vi "Power Meter Control Panel.vi"(8 "error in (no error)":errorcluster) -> (0 "error out":errorcluster)   [LabVIEW 2013]
doc: "(Dynamic) A user-level application that simulates the physical front panel of the Instrument. Provide the user with buttons to manually control features of the instrument, and provide indicators of its current state."
uses:
  Public/Filters.ctl
  <vilib>/Instr/_visa.llb/VISA Configure Serial Port (Instr).vi
  Newport 1830-C.lvlib
panel:
  in  "Baud rate (9600)":u32=115200
  out "Waveform Chart":dbl[unit](graph)=4.09e-07
  out "Sampling Rate":dbl
  in  "Which Filter":T1=1 items=["Orange"=1, "Green"=2, "Yellow"=3]
  out "Actual Power":dbl
  in  "Measured Power":dbl
  in  "Convert Power":bool
  in  "VISA Resource Name":refnum<visa-resource-name>="COM10"
  out "Initialized?":bool
  in  "Filter":T1=1 items=["Orange"=1, "Green"=2, "Yellow"=3]
  out "Power":string
  in  "Time between Reads (ms)":u32 max=1000 step=1
  in  "Read Continuous":bool
  in  "Averaging":u32=40 min=1 max=1024 step=1
  in  "Averaging":bool
  out "Units":u16(ring)=1 items=["W"=1, "dB"=2, "dBm"=3, "REL"=4]
  out "AVG":u16(ring)=2 items=["Slow"=1, "Medium"=2, "Fast"=3]
  out "Run/Stop":u16(ring) items=["Stop", "Run"]
  out "ATTN":u16(ring) items=["Off", "On"]
  out "Local Lockout":u16(ring) items=["Off", "On"]
  out "Zero":u16(ring) items=["Off", "On"]
  out "Beeper":u16(ring) items=["Off", "On"]
  out "Backlight":u16(ring) items=["Off", "Low", "High"]
  out "Range":u16(ring) items=["Auto", "Highest Sensitivity", "30uW", "300uW", "3mW", "30mW", "300mW", "3W", "Lowest Sensitivity"]
  in  "Run/Stop set":u32(ring)=1 items=["Stop", "Run"]
  in  "ATTN set":u32(ring) items=["Off", "On"]
  in  "BKLT set":u32(ring)=1 items=["Off", "Low", "High"]
  in  "Range set":u32(ring) items=["Auto", "Highest Sensitivity", "30uW", "300uW", "3mW", "30mW", "300mW", "3W", "Lowest Sensitivity"]
  in  "Beeper set":u32(ring) items=["Off", "On"]
  in  "AVG set":u32(ring)=2 items=["Slow"=1, "Medium"=2, "Fast"=3]
  in  "Units set":u32(ring)=1 items=["W"=1, "dB"=2, "mdB"=3, "REL"=4]
  in  "Zero set":u32(ring) items=["Off", "On"]
  in  "Local set":u32(ring) items=["Off", "On"]
  in  "Read Current Power":bool
  in  "Apply \nNew Settings":bool
  in  "Copy \nCurrent Settings\nto New Settings":bool
  in  "Read Settings":bool
  in  "Wavelength Set":dbl[unit]
  out "Wavelength":dbl[unit]
  in  "Copy actual to set":bool
  in  "Populate fields with member data":bool
  in  "stop":bool
  # "Newport 1830 Power Meter"
  # "New Settings"
  # "Current Settings"
  # "Convert Measured Power"
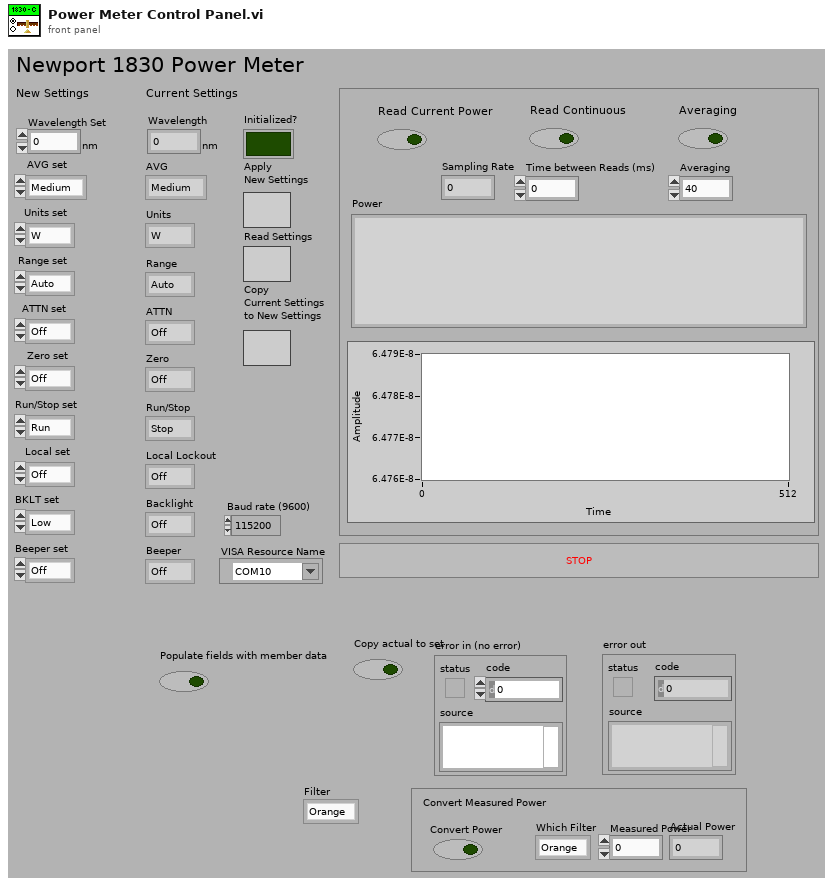
[diagram p1: front panel]
types:
  T1 = typedef "Newport 1830-C.lvlib/Filters.ctl" = u16
  T2 = cluster{"Wavelength":dbl[unit], "AVG":u16, "Range":u16, "Backlight":u16, "Beeper":u16, "Zero":u16, "Local Lockout":u16, "ATTN":u16, "Run/Stop":u16, "Units":u16, "Averaging Time":dbl, "Averaging":bool, "Most Recent Power":dbl, "Filter":T1}
  T3 = cluster{"Wavelength":dbl[unit], "AVG":u16, "Range":u16, "Backlight":u16, "Beeper":u16, "Zero":u16, "Local Lockout":u16, "ATTN":u16, "Run/Stop":u16, "Units":u16, "Averaging Points":u32, "Averaging":bool, "Most Recent Power":dbl, "Filter":T1}
  T4 = cluster{"Wavelength":dbl[unit], "AVG":i32, "Range":i32, "Backlight":i32, "Beeper":i32, "Zero":i32, "Local Lockout":i32, "ATTN":i32, "Run/Stop":i32, "Units":i32, "Averaging Points":u32, "Averaging":bool, "Most Recent Power":dbl, "Filter":i32}
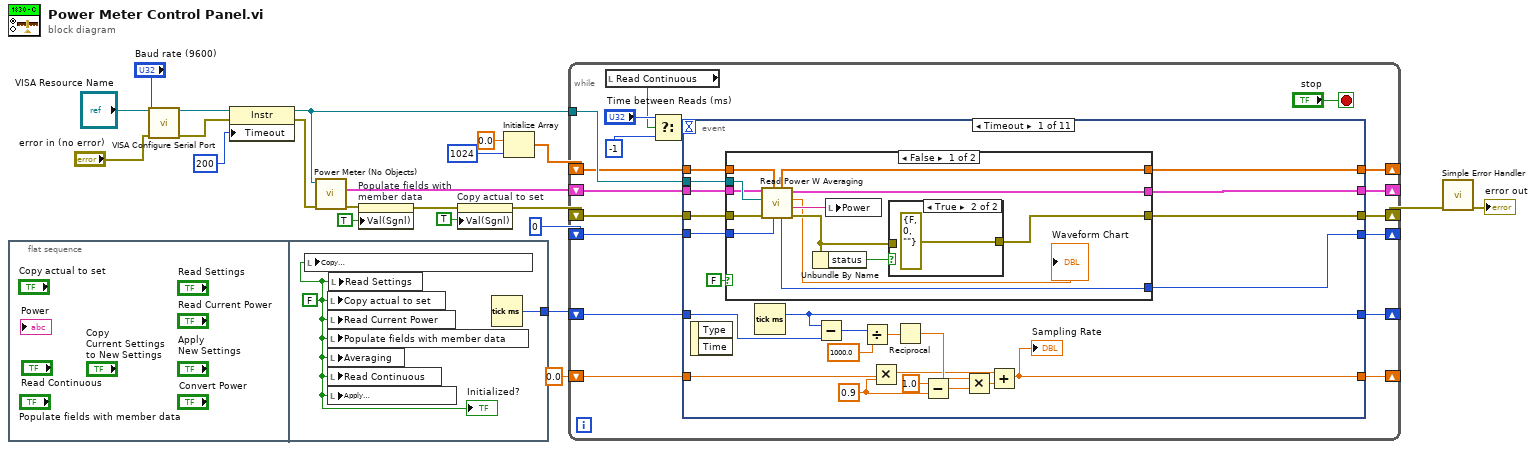
[diagram p0: block diagram]
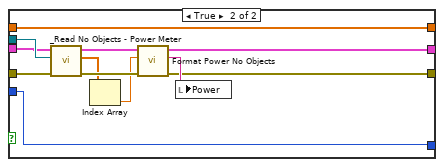
[diagram p3: hidden frame]
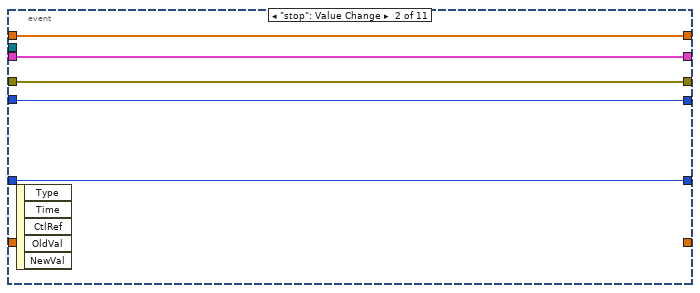
[diagram p4: hidden frame]
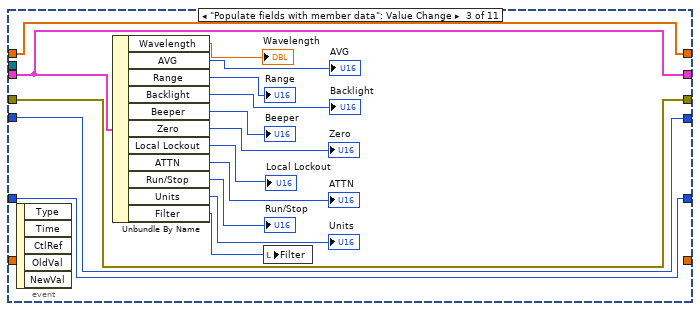
[diagram p5: hidden frame]
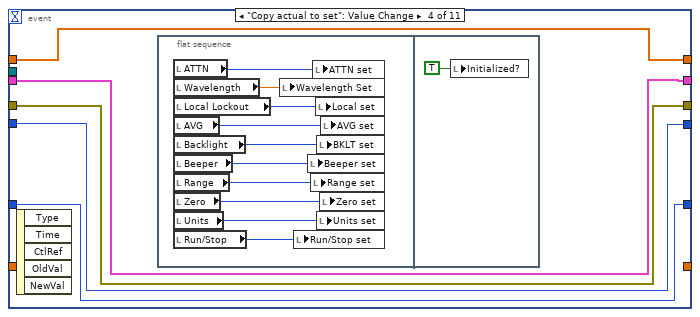
[diagram p6: hidden frame]
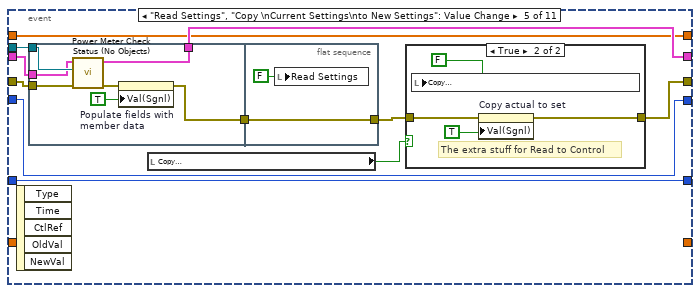
[diagram p7: hidden frame]
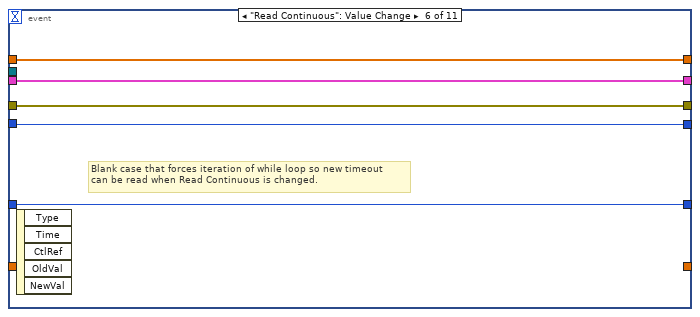
[diagram p9: hidden frame]
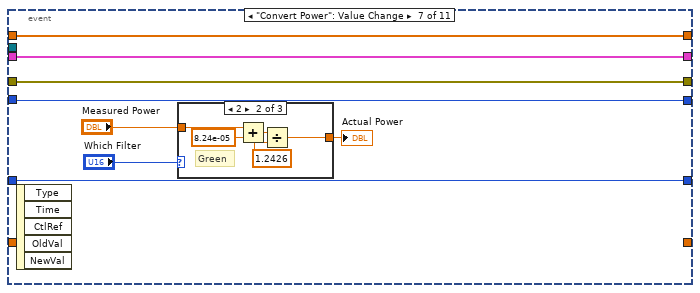
[diagram p10: hidden frame]
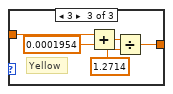
[diagram p12: hidden frame]
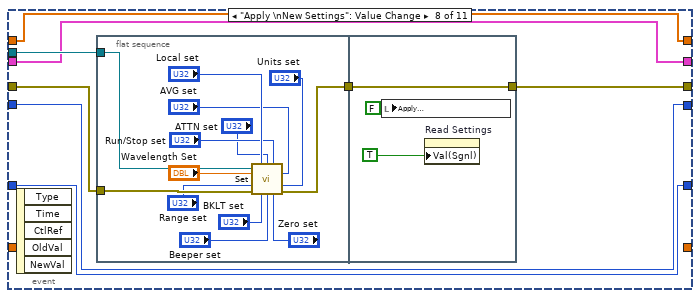
[diagram p13: hidden frame]
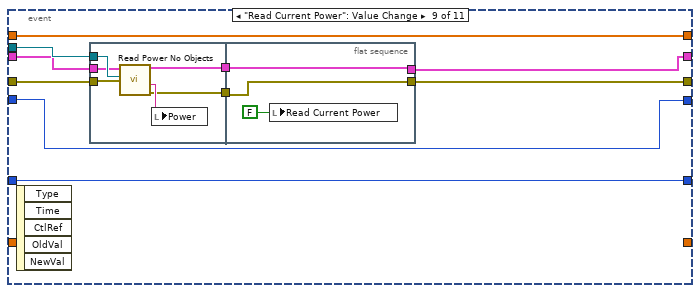
[diagram p14: hidden frame]
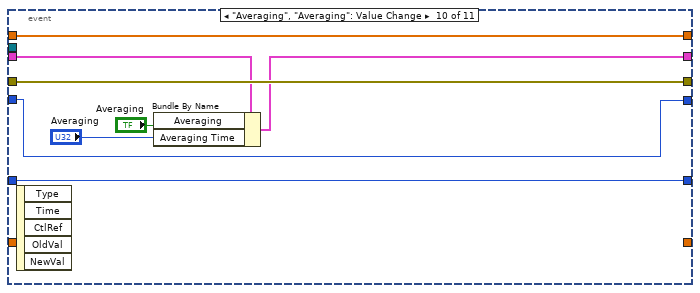
[diagram p15: hidden frame]
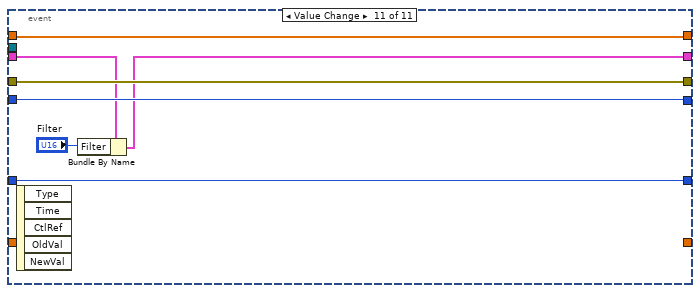
[diagram p16: hidden frame]
diagram:
  n1 = flat-sequence {
    tunnel: [w23] -> w3
    frame #0 {
    }
    frame #1 {
      w24 = FALSE ("Read")
      n2 = local write "Copy \nCurrent Settings\nto New Settings"(w24) -> ()
      n3 = local write "Copy actual to set"(w24) -> ()
      n4 = local write "Read Current Power"(w24) -> ()
      n5 = local write "Populate fields with member data"(w24) -> ()
      n6 = local write "Averaging"(w24) -> ()
      n7 = local write "Read Continuous"(w24) -> ()
      n8 = local write "Apply \nNew Settings"(w24) -> ()
      n9 = local write "Read Settings"(w24) -> ()
      n10 = Tick Count (ms)() -> (millisecond timer value=w23:u32)
      "Initialized?" <- w24
    }
  }
  n11 = call-poly "VISA Configure Serial Port"("VISA resource name"="VISA Resource Name", "baud rate (9600)"="Baud rate (9600)", "error in (no error)"="error in (no error)") -> ("VISA resource name out"=w8:refnum<visa-resource-name>, "error out"=w4:errorcluster)  [unwired: 7 in, 4 out]
  n12 = property class="Instr"(reference=w8, error in=w4, "Timeout"=u32 200 ("General Settings:Timeout Value")) -> (reference out=w9:refnum<visa-resource-name>, error out=w5:errorcluster)
  n13 = call "Power Meter (No Objects).vi"("error in (no error)"=w5, "VISA resource name"=w9) -> ("error out"=w16:errorcluster, "Power Meter Out"=w11:T2)  [unwired: 8 in]
  n14 = property on="Populate fields with member data" class="Bool (strict)"(error in=w16, "Val(Sgnl)"=TRUE ("Value (Signaling)")) -> (error out=w20:errorcluster)  [unwired: 1 in, 1 out]
  n15 = property on="Copy actual to set" class="Bool (strict)"(error in=w20, "Val(Sgnl)"=TRUE ("Value (Signaling)")) -> (error out=w19:errorcluster)  [unwired: 1 in, 1 out]
  n16 = Initialize Array(0.0 ("element"), 1024 ("dimension size")) -> (w13:dbl[])
  n17 = while {
    shift-right: [w41] -> _
    shift-left: w11 -> [w27]
    shift-right: [w40] -> w18
    shift-left: w19 -> [w42]
    tunnel: w9 -> [w37]
    shift-right: [w32] -> _
    shift-left: w13 -> [w33]
    shift-right: [w30] -> _
    shift-left: 0 -> [w31]
    shift-right: [w29] -> _
    shift-left: w3 -> [w28]
    shift-right: [w26] -> _
    shift-left: 0.0 -> [w25]
    stop <- "stop" stop-if-true
    n18 = local read "Read Continuous"() -> (w35:bool)
    n19 = Select(t="Time between Reads (ms)", s=w35, f=-1) -> (s? t:f=w38:u32)
    n20 = event shown="[0] Timeout" {
      selector: _ -> [_ _ _ _ _ _ _ _ _ _ _]
      dyn-events: _ -> [_ _ _ _ _ _ _ _ _ _ _]
      timeout: w38 -> [_ _ _ _ _ _ _ _ _ _ _]
      tunnel: [w61 w94 w98 w114 w135 w157 w160 w179 w207 w224 w230] -> w41
      tunnel: [w64 w97 w112 w118 w136 w159 w167 w185 w209 w229 w235] -> w40
      tunnel: w42 -> [w65 w97 w112 w118 w140 w159 w167 w186 w211 w229 w235]
      tunnel: w37 -> [w63 _ _ _ w134 _ _ w184 w208 _ _]
      tunnel: w33 -> [w60 w96 w101 w117 w133 w158 w163 w182 w206 w226 w234]
      tunnel: [w59 w96 w101 w117 w133 w158 w163 w182 w206 w226 w234] -> w32
      tunnel: w31 -> [w58 w93 w99 w116 w131 w155 w161 w180 w204 w222 w232]
      tunnel: [w57 w93 w99 w116 w131 w155 w161 w180 w204 w222 w232] -> w30
      tunnel: [w55 w95 w100 w115 w130 w156 w162 w181 w203 w223 w233] -> w29
      tunnel: w28 -> [w56 w95 w100 w115 w130 w156 w162 w181 w203 w223 w233]
      tunnel: w27 -> [w52 w94 w98 w114 w132 w157 w160 w179 w205 w225 w231]
      tunnel: [w43 _ _ _ _ _ _ _ _ _ _] -> w26
      tunnel: w25 -> [w51 _ _ _ _ _ _ _ _ _ _]
      event Timeout {
        w48 = 0.9 ("y")
        n21 = event-data() -> ()  [unwired: 1 in, 2 out]
        n22 = case shown="False" FALSE {
          tunnel: w65 -> [w77 w92]
          tunnel: [w72 w87] -> w64
          tunnel: [w76 w86] -> w61
          tunnel: w63 -> [w78 w85]
          tunnel: w60 -> [w71 w83]
          tunnel: [w70 w83] -> w59
          tunnel: w58 -> [w69 w82]
          tunnel: [w68 w82] -> w57
          tunnel: w52 -> [w66 w81]
          frame False {
            n23 = call "Read Power W Averaging.vi"("Index In"=w69, "Buffer In"=w71, "error in (no error)"=w77, "VISA Resource Name"=w78, "Cluster In"=w66) -> ("error out"=w74:errorcluster, "Current Power w/ Units"=w75:string, "Current Power"=→"Waveform Chart":dbl[unit], "Cluster Out"=w76:T3, "Index Out"=w68:u32, "Buffer Out"=w70:dbl[])  [unwired: 1 in]
            n24 = Unbundle By Name(w74) -> ("status"=w73:bool)
            n25 = local write "Power"(w75) -> ()
            n26 = case shown="True" w73 {
              tunnel: w74 -> [w79 _]
              tunnel: [w79 errorcluster {"status"=FALSE, "code"=0, "source"=""} ("error out")] -> w72
              frame False {
              }
              frame True {
              }
            }
          }
          frame True {
            n27 = call "_Read No Objects - Power Meter.vi"("error in (no error)"=w92, "VISA Resource Name In"=w85, "Power Meter in"=w81) -> ("error out"=w91:errorcluster, "X array"=w90:dbl[], "Power Meter Out"=w84:T4)  [unwired: 5 in, 1 out]
            n28 = Index Array(array=w90) -> (element=w89:dbl)  [unwired: 1 in]
            n29 = call "Format Power No Objects.vi"("error in"=w91, "Power"=w89, "Cluster In"=w84) -> ("error out"=w87:errorcluster, "Formatted Power"=w88:string, "Cluster Out"=w86:T3)  [unwired: 6 in]
            n30 = local write "Power"(w88) -> ()
          }
        }
        n31 = Tick Count (ms)() -> (millisecond timer value=w55:u32)
        n32 = Subtract(x=w55, y=w56) -> (x-y=w54:u32)
        n33 = Divide(x=w54, y=1000.0) -> (x/y=w53:dbl)
        n34 = Multiply(x=w51, y=w48) -> (x*y=w44:dbl)
        n35 = Reciprocal(x=w53) -> (1/x=w50:dbl)
        n36 = Subtract(x=1.0, y=w48) -> (x-y=w46:dbl)
        n37 = Multiply(x=w50, y=w46) -> (x*y=w45:dbl)
        n38 = Add(x=w44, y=w45) -> (x+y=w43:dbl)
        "Sampling Rate" <- w43
      }
      event "stop": Value Change {
        n39 = event-data() -> ()  [unwired: 1 in, 5 out]
      }
      event "Populate fields with member data": Value Change {
        n40 = event-data() -> ()  [unwired: 1 in, 5 out]
        n41 = Unbundle By Name(w98) -> ("Wavelength"=→"Wavelength":dbl[unit], "AVG"=→"AVG":u16, "Range"=→"Range":u16, "Backlight"=→"Backlight":u16, "Beeper"=→"Beeper":u16, "Zero"=→"Zero":u16, "Local Lockout"=→"Local Lockout":u16, "ATTN"=→"ATTN":u16, "Run/Stop"=→"Run/Stop":u16, "Units"=→"Units":u16, "Filter"=w102:T1)
        n42 = local write "Filter"(w102) -> ()
      }
      event "Copy actual to set": Value Change {
        n43 = event-data() -> ()  [unwired: 1 in, 5 out]
        n44 = flat-sequence {
          frame #0 {
            n45 = local read "ATTN"() -> (w120:u16)
            n46 = local read "Wavelength"() -> (w128:dbl[unit])
            n47 = local read "Local Lockout"() -> (w124:u16)
            n48 = local read "AVG"() -> (w127:u16)
            n49 = local read "Backlight"() -> (w126:u16)
            n50 = local read "Beeper"() -> (w125:u16)
            n51 = local read "Range"() -> (w123:u16)
            n52 = local read "Zero"() -> (w119:u16)
            n53 = local read "Units"() -> (w121:u16)
            n54 = local read "Run/Stop"() -> (w122:u16)
            n55 = local write "Wavelength Set"(w128) -> ()
            n56 = local write "Run/Stop set"(w122) -> ()
            n57 = local write "Beeper set"(w125) -> ()
            n58 = local write "Range set"(w123) -> ()
            n59 = local write "ATTN set"(w120) -> ()
            n60 = local write "Local set"(w124) -> ()
            n61 = local write "BKLT set"(w126) -> ()
            n62 = local write "Units set"(w121) -> ()
            n63 = local write "Zero set"(w119) -> ()
            n64 = local write "AVG set"(w127) -> ()
          }
          frame #1 {
            n65 = local write "Initialized?"(TRUE ("Power\nMeter\nInitialized?")) -> ()
          }
        }
      }
      event "Read Settings", "Copy \nCurrent Settings\nto New Settings": Value Change {
        n66 = event-data() -> ()  [unwired: 1 in, 5 out]
        n67 = flat-sequence {
          tunnel: w140 -> [w152]
          tunnel: [w149] -> w137
          tunnel: [w151] -> w135
          tunnel: w134 -> [w147]
          tunnel: w132 -> [w146]
          tunnel: [w153] -> w138
          tunnel: w137 -> [w153]
          frame #0 {
            n68 = call "Power Meter Check Status (No Objects).vi"("error in (no error)"=w152, "VISA resource name"=w147, "Cluster In"=w146) -> ("error out"=w150:errorcluster, "Cluster Out"=w151:T3)  [unwired: 6 in, 1 out]
            n69 = property on="Populate fields with member data" class="Bool (strict)"(error in=w150, "Val(Sgnl)"=TRUE ("Value (Signaling)")) -> (error out=w149:errorcluster)  [unwired: 1 in, 1 out]
          }
          frame #1 {
            n70 = local write "Read Settings"(FALSE ("Read")) -> ()
          }
        }
        n71 = local read "Copy \nCurrent Settings\nto New Settings"() -> (w139:bool)
        n72 = case shown="True" w139 {
          tunnel: w138 -> [w141 w143]
          tunnel: [w141 w142] -> w136
          frame False {
          }
          frame True {
            # "The extra stuff for Read to Control"
            n73 = local write "Copy \nCurrent Settings\nto New Settings"(FALSE ("Read")) -> ()
            n74 = property on="Copy actual to set" class="Bool (strict)"(error in=w143, "Val(Sgnl)"=TRUE ("Value (Signaling)")) -> (error out=w142:errorcluster)  [unwired: 1 in, 1 out]
          }
        }
      }
      event "Read Continuous": Value Change {
        # "Blank case that forces iteration of while loop so new timeout\ncan be read when Read Continuous is changed."
        n75 = event-data() -> ()  [unwired: 1 in, 5 out]
      }
      event "Convert Power": Value Change {
        n76 = event-data() -> ()  [unwired: 1 in, 5 out]
        n77 = case shown="2" "Which Filter" {
          tunnel: "Measured Power" -> [w168 w170 w175]
          tunnel: [w168 w169 w174] -> w165
          frame 1, Default {
            # "Orange"
          }
          frame 2 {
            # "Green"
            n78 = Add(x=w170, y=8.24e-05) -> (x+y=w171:dbl)
            n79 = Divide(x=w171, y=1.2426) -> (x/y=w169:dbl)
          }
          frame 3 {
            # "Yellow"
            n80 = Add(x=w175, y=0.0001954) -> (x+y=w176:dbl)
            n81 = Divide(x=w176, y=1.2714) -> (x/y=w174:dbl)
          }
        }
        "Actual Power" <- w165
      }
      event "Apply \nNew Settings": Value Change {
        n82 = event-data() -> ()  [unwired: 1 in, 5 out]
        n83 = flat-sequence {
          tunnel: w186 -> [w198]
          tunnel: w184 -> [w199]
          tunnel: [w187] -> w183
          tunnel: [w200] -> w185
          tunnel: w183 -> [w200]
          frame #0 {
            n84 = call "Set.vi"("VISA resource name"=w199, "Local Lockout (0:1)"="Local set", "ATTN (0:1)"="ATTN set", "Run/Stop (1:0)"="Run/Stop set", "Wavelength (nnnn)"="Wavelength Set", "AVG (1:3)"="AVG set", "Range (0-Auto,1:8)"="Range set", "Units (1:4)"="Units set", "error in (no error)"=w198, "Backlight (0:2)"="BKLT set", "Beeper (0:1)"="Beeper set", "Zero (0:1)"="Zero set") -> ("error out"=w187:errorcluster)  [unwired: 2 in, 1 out]
          }
          frame #1 {
            n85 = local write "Apply \nNew Settings"(FALSE ("Set")) -> ()
            n86 = property on="Read Settings" class="Bool (strict)"("Val(Sgnl)"=TRUE ("Value (Signaling)")) -> ()  [unwired: 2 in, 2 out]
          }
        }
      }
      event "Read Current Power": Value Change {
        n87 = event-data() -> ()  [unwired: 1 in, 5 out]
        n88 = flat-sequence {
          tunnel: [w215] -> w212
          tunnel: w211 -> [w218]
          tunnel: [w216] -> w210
          tunnel: w208 -> [w214]
          tunnel: w205 -> [w213]
          tunnel: [w220] -> w207
          tunnel: w212 -> [w220]
          tunnel: [w219] -> w209
          tunnel: w210 -> [w219]
          frame #0 {
            n89 = call "Read Power No Objects.vi"("error in (no error)"=w218, "VISA Resource Name"=w214, "Cluster In"=w213) -> ("error out"=w216:errorcluster, "Current Power w/ Units"=w217:string, "Cluster Out"=w215:T3)  [unwired: 5 in, 1 out]
            n90 = local write "Power"(w217) -> ()
          }
          frame #1 {
            n91 = local write "Read Current Power"(FALSE ("Read Current Value")) -> ()
          }
        }
      }
      event "Averaging", "Averaging": Value Change {
        n92 = event-data() -> ()  [unwired: 1 in, 5 out]
        n93 = Bundle By Name(cluster=w225, "Averaging"="Averaging", "Averaging Time"="Averaging") -> (w224:T2)
      }
      event Value Change {
        n94 = event-data() -> ()  [unwired: 1 in, 5 out]
        n95 = Bundle By Name(cluster=w231, "Filter"="Filter") -> (w230:T2)
      }
    }
  }
  n96 = call <vilib>:"Simple Error Handler.vi"("error in (no error)"=w18) -> ("error out"=→"error out":errorcluster)  [unwired: 1 in, 7 out]
